vi "SMSAlert.vi"(0 "Send Message?":bool, 1 "Error Message to be sent":string, 2 "Vehicle":string, 9 "Error Alarm?":bool, 11 "Soft Alarm?":bool, 12 "Recipients":string[](array[string])) -> ()   [LabVIEW 2014]
uses:
  C:/Users/V4/Desktop/OMEGA/Windows/SubVIs Win/SMS_Alert/SMSmk3.dll
  SMSmk3.dll
panel:
  out "Sent To":string[](array[string])
  out "Person(s) to send to":string[](array[string])
  out "Names in CSV file":string[](array[string])
  out "Contacts Error":errorcluster
  out "Numbers to be messaged":string[](array[string])
  out "Send Message Error":errorcluster
  out "Name And Number":string
  in  "Index":i32
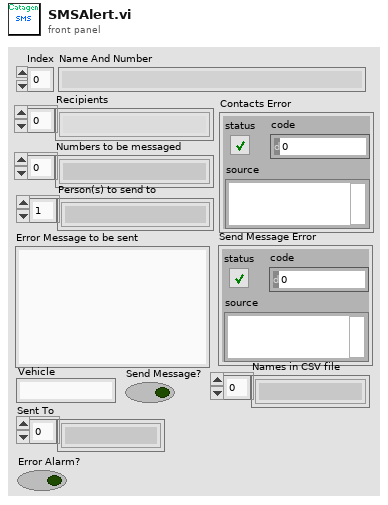
[diagram p1: front panel]
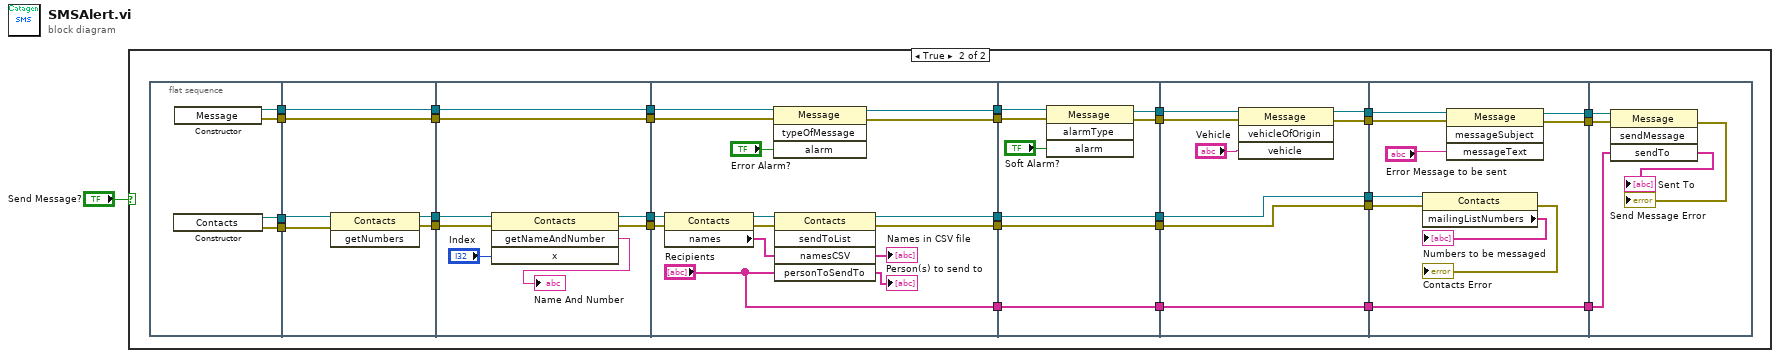
[diagram p0: block diagram]
diagram:
  n1 = case shown="True" "Send Message?" {
    frame False {
    }
    frame True {
      n2 = flat-sequence {
        tunnel: [w35] -> w31
        tunnel: [w34] -> w30
        tunnel: [w32] -> w29
        tunnel: [w33] -> w28
        tunnel: w31 -> [w37]
        tunnel: w30 -> [w36]
        tunnel: [w37] -> w27
        tunnel: [w36] -> w26
        tunnel: w29 -> [w41]
        tunnel: w28 -> [w40]
        tunnel: [w39] -> w25
        tunnel: [w38] -> w24
        tunnel: w27 -> [w43]
        tunnel: w26 -> [w42]
        tunnel: [w43] -> w23
        tunnel: [w42] -> w22
        tunnel: w25 -> [w47]
        tunnel: w24 -> [w46]
        tunnel: [w45] -> w21
        tunnel: [w44] -> w20
        tunnel: w23 -> [w54]
        tunnel: w22 -> [w53]
        tunnel: [w52] -> w19
        tunnel: [w51] -> w18
        tunnel: w21 -> [w64]
        tunnel: [w59] -> w17
        tunnel: w20 -> [w63]
        tunnel: [w58] -> w16
        tunnel: ["Recipients"] -> w2
        tunnel: w19 -> [w71]
        tunnel: w18 -> [w70]
        tunnel: [w69] -> w15
        tunnel: [w68] -> w14
        tunnel: w17 -> [w67]
        tunnel: w16 -> [w66]
        tunnel: [w66] -> w13
        tunnel: [w67] -> w8
        tunnel: [w65] -> w3
        tunnel: w2 -> [w65]
        tunnel: w15 -> [w78]
        tunnel: w14 -> [w77]
        tunnel: [w79] -> w12
        tunnel: [w80] -> w11
        tunnel: w13 -> [w75]
        tunnel: w8 -> [w74]
        tunnel: [w75] -> w7
        tunnel: [w74] -> w6
        tunnel: [w73] -> w4
        tunnel: w3 -> [w73]
        tunnel: w12 -> [w86]
        tunnel: w11 -> [w89]
        tunnel: [w88] -> w10
        tunnel: [w87] -> w9
        tunnel: w7 -> [w83]
        tunnel: w6 -> [w82]
        tunnel: [w81] -> w5
        tunnel: w4 -> [w81]
        tunnel: w10 -> [w94]
        tunnel: w9 -> [w93]
        tunnel: w5 -> [w92]
        frame #0 {
          n3 = constructor class="Contacts"() -> (reference out=w33:refnum<k24>, error out=w32:errorcluster)  [unwired: 3 in, 1 out]
          n4 = constructor class="Message"() -> (reference out=w35:refnum<k24>, error out=w34:errorcluster)  [unwired: 3 in, 1 out]
        }
        frame #1 {
          n5 = invoke class="Contacts" method="getNumbers"(reference=w40, error in=w41) -> (reference out=w39:refnum<k24>, error out=w38:errorcluster)  [unwired: 1 in, 1 out]
        }
        frame #2 {
          n6 = invoke class="Contacts" method="getNameAndNumber"(reference=w47, error in=w46, "x"="Index") -> (reference out=w45:refnum<k24>, error out=w44:errorcluster, "getNameAndNumber"=→"Name And Number":string)  [unwired: 1 in, 1 out]
        }
        frame #3 {
          n7 = property class="Contacts"(reference=w64, error in=w63) -> (reference out=w62:refnum<k24>, error out=w61:errorcluster, "names"=w60:string[])
          n8 = invoke class="Message" method="typeOfMessage"(reference=w54, error in=w53, "alarm"="Error Alarm?") -> (reference out=w52:refnum<k24>, error out=w51:errorcluster)  [unwired: 1 in, 2 out]
          n9 = invoke class="Contacts" method="sendToList"(reference=w62, error in=w61, "namesCSV"=w60, "personToSendTo"="Recipients") -> (reference out=w59:refnum<k24>, error out=w58:errorcluster, "namesCSV"=→"Names in CSV file":string[], "personToSendTo"=→"Person(s) to send to":string[])  [unwired: 1 in, 1 out]
        }
        frame #4 {
          n10 = invoke class="Message" method="alarmType"(reference=w71, error in=w70, "alarm"="Soft Alarm?") -> (reference out=w69:refnum<k24>, error out=w68:errorcluster)  [unwired: 1 in, 2 out]
        }
        frame #5 {
          n11 = invoke class="Message" method="vehicleOfOrigin"(reference=w78, error in=w77, "vehicle"="Vehicle") -> (reference out=w79:refnum<k24>, error out=w80:errorcluster)  [unwired: 1 in, 2 out]
        }
        frame #6 {
          n12 = property class="Contacts"(reference=w82, error in=w83) -> (error out=→"Contacts Error":errorcluster, "mailingListNumbers"=→"Numbers to be messaged":string[])  [unwired: 1 out]
          n13 = invoke class="Message" method="messageSubject"(reference=w86, error in=w89, "messageText"="Error Message to be sent") -> (reference out=w88:refnum<k24>, error out=w87:errorcluster)  [unwired: 1 in, 2 out]
        }
        frame #7 {
          n14 = invoke class="Message" method="sendMessage"(reference=w94, error in=w93, "sendTo"=w92) -> (error out=→"Send Message Error":errorcluster, "sendTo"=→"Sent To":string[])  [unwired: 1 in, 2 out]
        }
      }
    }
  }
